vi "Close.vi"(8 "error in (no error)":errorcluster, 11 "reference in":refnum<class "Switch_MotorP5.lvclass">) -> (0 "error out":errorcluster, 3 "reference in":refnum<class "Switch_MotorP5.lvclass">)   [LabVIEW 2022 SP3, in "Switch_MotorP5.lvlib" / "Switch_MotorP5.lvclass"]
uses:
  Switch_MotorP5.lvclass
  Components/SwitchBase.lvlibp/SwitchBase.lvclass
  Components/ViPER.lvlibp/ViPER.lvclass
  C:/Projects/Medulla/ViPER/Examples/Flux_Capacitor_Tester/Components/ViPER.lvlibp/ViPER.lvclass
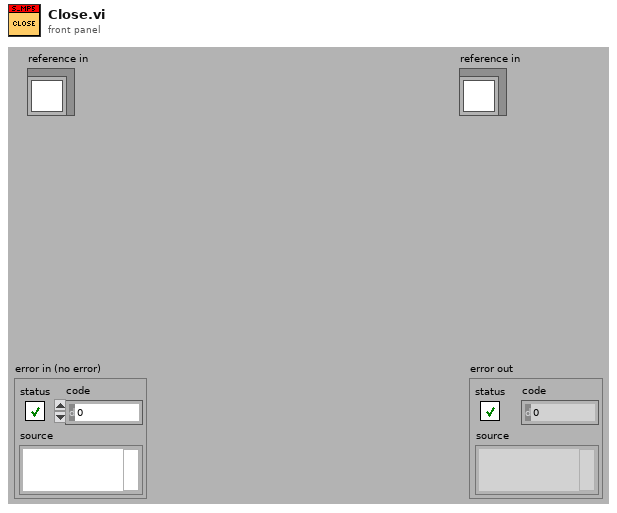
[diagram p1: front panel]
types:
  T1 = typedef "Switch_MotorP5.lvlib/Switch_MotorP5.lvclass/ObjectAttributes.ctl" = cluster{"Config":T2, "VISA":refnum<visa-resource-name>, "RPM":i32, "States":bool[], "UpdateEvent":refnum<user-event>, "Motor":enum32{"M1", "M2", "M3", "M4", "M5", "M6", "M7", "M8"}}
  T2 = typedef "Switch_MotorP5.lvlib/Switch_MotorP5.lvclass/Config.ctl" = cluster{"COM":refnum<visa-resource-name>, "SwitchMap":cluster{"Name":string, "Description":string, "Group":string, "IsGroup":bool, "Motor":enum32{"M1", "M2", "M3", "M4", "M5", "M6", "M7", "M8", "NA"}}[], "Sim":bool}
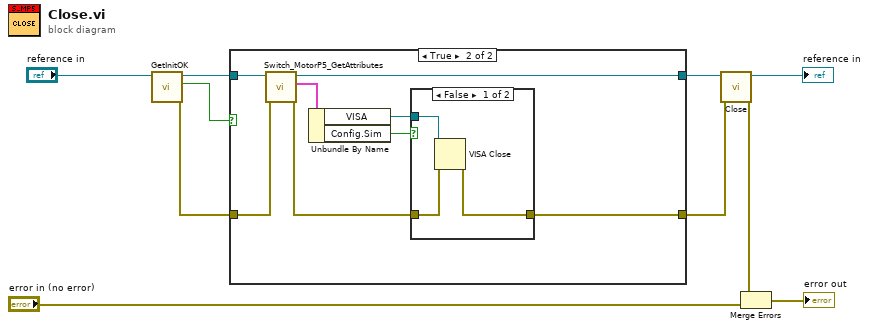
[diagram p0: block diagram]
diagram:
  n1 = call "GetInitOK.vi"("reference in"="reference in") -> ("error out"=w4:errorcluster, "init_ok"=w5:bool, "reference out"=w6:refnum<class "Switch_MotorP5.lvclass">)  [unwired: 8 in]
  n2 = case shown="True" w5 {
    tunnel: w4 -> [w12 w19]
    tunnel: [w12 w15] -> w7
    tunnel: w6 -> [w11 w20]
    tunnel: [w11 w18] -> w8
    frame False {
    }
    frame True {
      n3 = call "Switch_MotorP5_GetAttributes.vi"("error in (no error)"=w19, "reference in"=w20) -> ("error out"=w16:errorcluster, "Data"=w17:T1, "reference out"=w18:refnum<class "Switch_MotorP5.lvclass">)  [unwired: 6 in, 1 out]
      n4 = Unbundle By Name(w17) -> ("VISA"=w14:refnum<visa-resource-name>, "Config.Sim"=w13:bool)
      n5 = case shown="False" w13 {
        tunnel: w16 -> [w23 w24]
        tunnel: [w22 w24] -> w15
        tunnel: w14 -> [w21 _]
        frame False {
          n6 = VISA Close(VISA resource name=w21, error in (no error)=w23) -> (error out=w22:errorcluster)
        }
        frame True {
        }
      }
    }
  }
  n7 = call-parent "Close.vi"("error in (no error)"=w7, "reference in"=w8) -> ("error out"=w3:errorcluster, "reference in"=→"reference in":refnum<class "Switch_MotorP5.lvclass">)  [unwired: 8 in]
  n8 = Merge Errors(w3, "error in (no error)") -> (→"error out":errorcluster)
